vi "Length Encoded String.vi"(0 "Bytes in":u8[](array[numeric]), 11 "Start Index(0)":i32) -> (4 "Remaining Bytes out":u8[](array[numeric]), 6 "String Bytes":u8[](array[numeric]), 8 "String":string, 10 "Length":i32, 15 "End Index":i32)   [LabVIEW 2014, in "hse-db.lvlib" / "MySQL (TCP).lvlib"]
uses:
  MySQL (TCP).lvlib
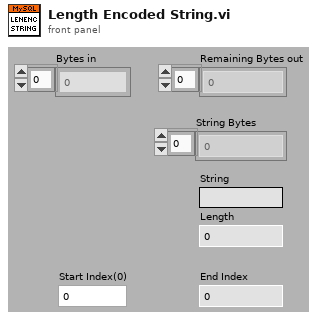
[diagram p1: front panel]
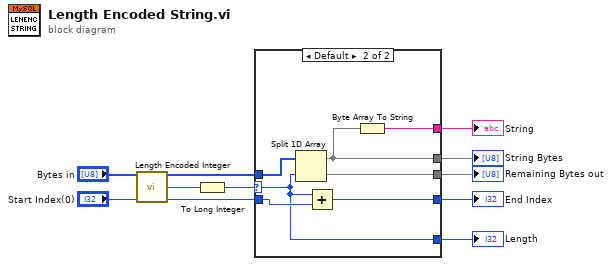
[diagram p0: block diagram]
diagram:
  n1 = call "Length Encoded Integer.vi"("Bytes in"="Bytes in", "Start Index(0)"="Start Index(0)") -> ("Remaining Bytes out"=w6:u8[], "Integer"=w3:u64, "End Index"=w7:i32)  [unwired: 10 in, 1 out]
  n2 = To Long Integer(number=w3) -> (32bit integer=w2:i32)
  n3 = case shown="Default" w2 {
    selector: w2 -> [_ w17]
    tunnel: [_ w14] -> w11
    tunnel: w6 -> [w12 w18]
    tunnel: [w13 w20] -> w10
    tunnel: w7 -> [w13 w19]
    tunnel: [_ w15] -> w9
    tunnel: [_ w17] -> w4
    tunnel: [w12 w16] -> w1
    frame 251 {
      # "NULL"
    }
    frame Default {
      n4 = Split 1D Array(array=w18, index=w17) -> (first subarray=w15:u8[], second subarray=w16:u8[])
      n5 = Add(x=w17, y=w19) -> (x+y=w20:i32)
      n6 = Byte Array To String(unsigned byte array=w15) -> (string=w14:string)
    }
  }
  "String" <- w11
  "End Index" <- w10
  "Remaining Bytes out" <- w1
  "String Bytes" <- w9
  "Length" <- w4
